vi "Destructor.vi"(8 "ErrorIn":errorcluster, 11 "TAFTraceWindow in":refnum<class "TAFTraceWindow.lvclass">) -> (0 "ErrorOut":errorcluster, 3 "TAFTraceWindow out":refnum<class "TAFTraceWindow.lvclass">)   [LabVIEW 2021, in "TAFTraceWindow.lvclass"]
uses:
  TAFTraceWindow.lvclass
  C:/Localdata/Projects/TriekselSoft/TriekselsoftApplicationFramework/Source/.Externals/Library_YAF/YActor/YActor.lvclass
  TAFTraceWindow.lvclass/TAFTraceWindow.ctl
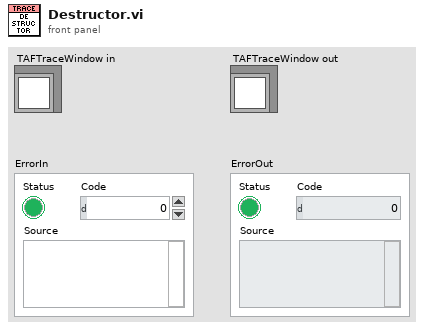
[diagram p1: front panel]
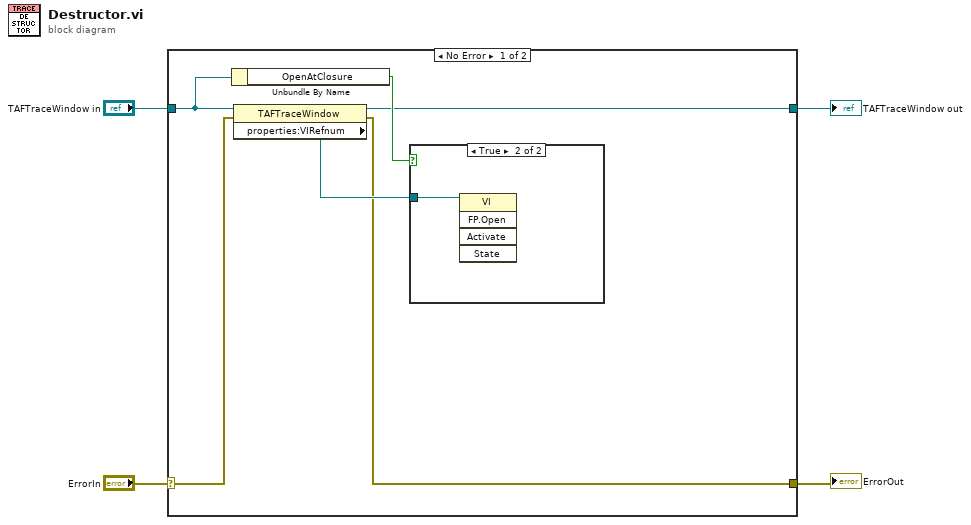
[diagram p0: block diagram]
diagram:
  n1 = case shown="No Error" "ErrorIn" {
    selector: "ErrorIn" -> [w6 w13]
    tunnel: [w5 w13] -> w3
    tunnel: [w8 w12] -> w1
    tunnel: "TAFTraceWindow in" -> [w10 w12]
    frame No Error {
      n2 = Unbundle By Name(w10) -> ("OpenAtClosure"=w9:bool)
      n3 = property class="TAFTraceWindow"(reference=w10, error in=w6) -> (reference out=w8:refnum<class "TAFTraceWindow.lvclass">, error out=w5:errorcluster, "properties:VIRefnum"=w7:refnum<vi>)
      n4 = case shown="True" w9 {
        tunnel: w7 -> [_ w11]
        frame False {
        }
        frame True {
          n5 = invoke class="VI" method="FP.Open"(reference=w11) -> ()  [unwired: 4 in, 5 out]
        }
      }
    }
    frame Error {
    }
  }
  "ErrorOut" <- w3
  "TAFTraceWindow out" <- w1
